vi "Block_No_Av.vi"(2 "Desired Averaging Time (mins)":dbl=5.0, 3 "Raw data file":path, 4 "Results file":path) -> ()   [LabVIEW 2022 SP3]
uses:
  Controls/Post_Process.ctl
  Controls/Setup.ctl
  Controls/Save_Data.ctl
  Globals/Meas_global.vi
  Block_Control_global.vi
  Globals/Dynamic_call_global.ph.vi
panel:
  out "Current Row Number":i32
  out "No of Rows":i32
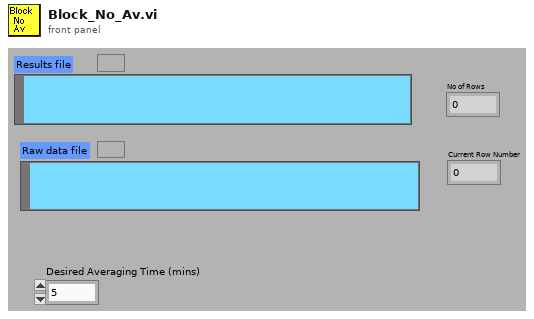
[diagram p1: front panel]
types:
  T1 = typedef "Save_Data.ctl" = enum16{"Save No Data", "Save Data"}
  T2 = typedef "Setup.ctl" = enum16{"Run Program", "Show Setup", "Save Current Setup", "Setup Front Panel"}
  T3 = typedef "Post_Process.ctl" = enum16{"Take New Data", "Post Process Raw Data File"}
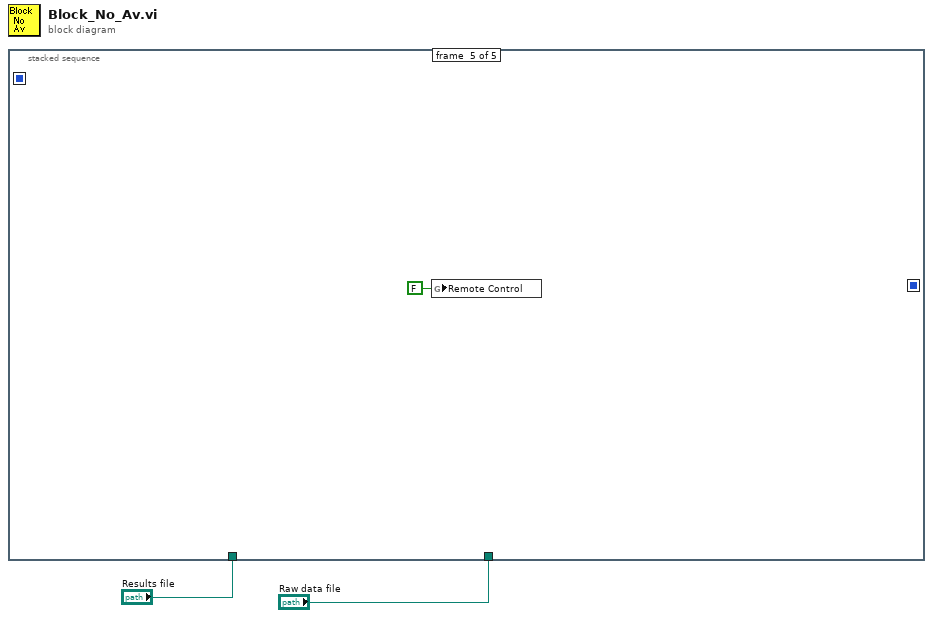
[diagram p0: block diagram]
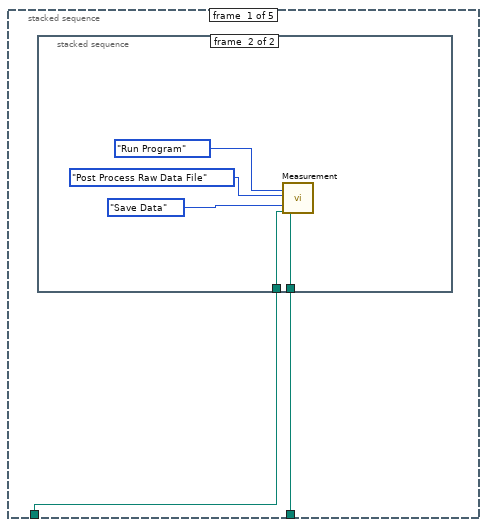
[diagram p2: hidden frame]
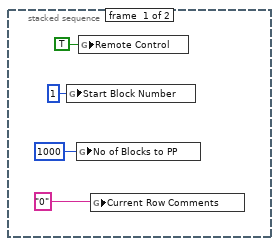
[diagram p3: hidden frame]
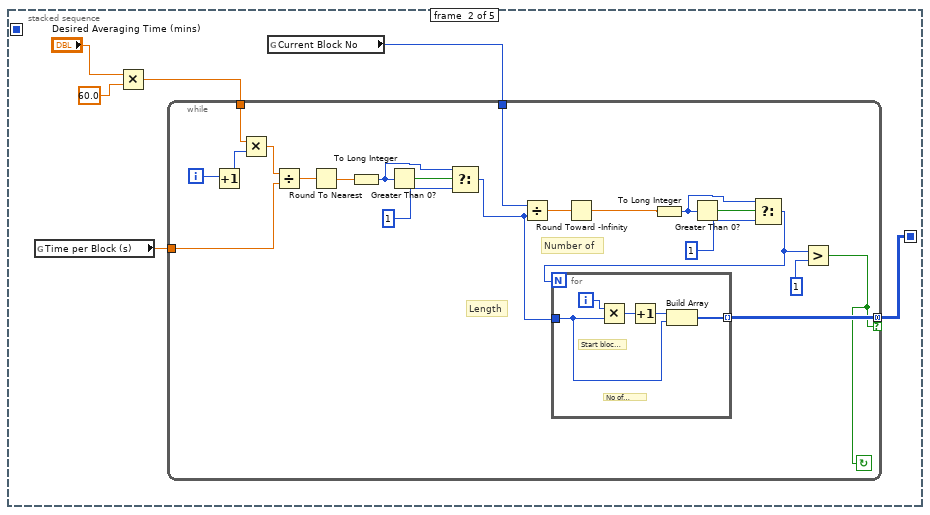
[diagram p4: hidden frame]
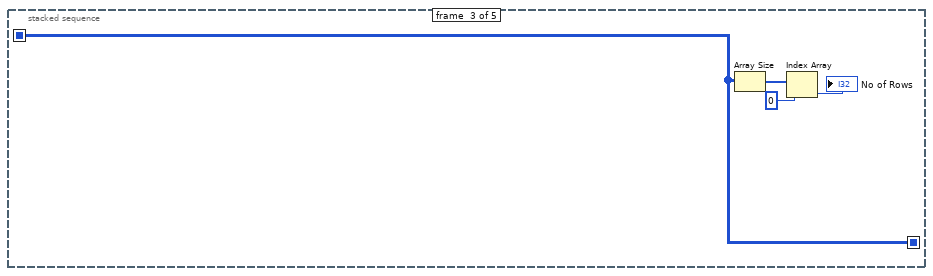
[diagram p5: hidden frame]
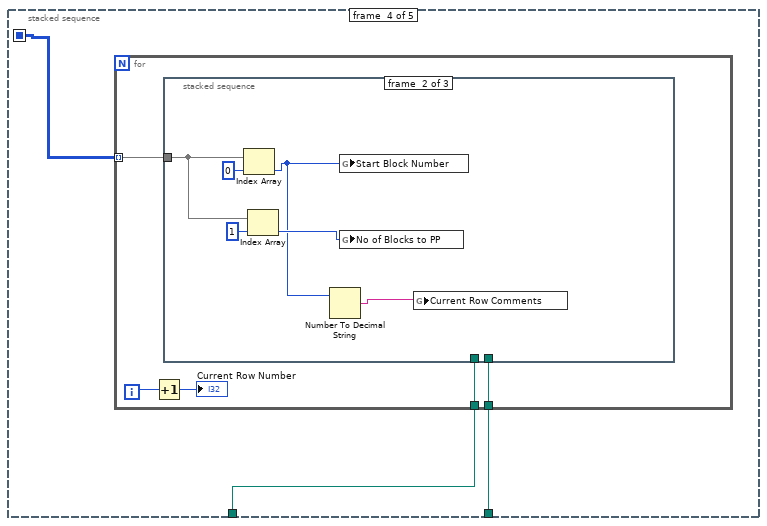
[diagram p6: hidden frame]
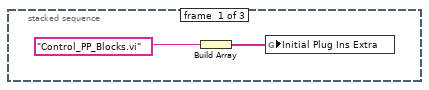
[diagram p7: hidden frame]
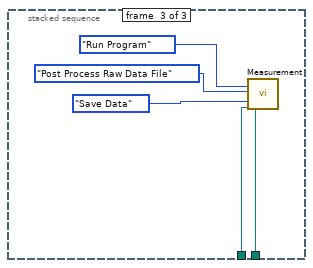
[diagram p8: hidden frame]
diagram:
  n1 = stacked-sequence {
    seq-local: [_ _ w46 _ _] -> [_ _ _ w50 _]
    seq-local: [_ w14 _ _ _] -> [_ _ w46 _ _]
    tunnel: "Raw data file" -> [w4 _ _ w52 _]
    tunnel: "Results file" -> [w3 _ _ w51 _]
    frame #0 {
      n2 = stacked-sequence {
        tunnel: w4 -> [_ w11]
        tunnel: w3 -> [_ w10]
        frame #0 {
          n3 = global write "Block_Control_global.vi" "Start Block Number"(1 ("Start Block Number")) -> ()
          n4 = global write "Block_Control_global.vi" "No of Blocks to PP"(1000 ("Start Block Number")) -> ()
          n5 = global write "Block_Control_global.vi" "Remote Control"(TRUE ("Remote Control")) -> ()
          n6 = global write "Meas_global.vi" "Current Row Comments"("0") -> ()
        }
        frame #1 {
          n7 = call "Measurement.vi"("setup"=Setup."Run Program", "Post Process"=Post_Process."Post Process Raw Data File", "File"=Save_Data."Save Data", "Results file"=w10, "Raw data file"=w11) -> ()  [unwired: 1 in, 14 out]
        }
      }
    }
    frame #1 {
      n8 = global read "Meas_global.vi" "Time per Block (s)"() -> (w18:dbl)
      n9 = Multiply(x="Desired Averaging Time (mins)", y=60.0) -> (x*y=w15:dbl)
      n10 = global read "Meas_global.vi" "Current Block No"() -> (w19:i32)
      n11 = while {
        tunnel: w19 -> [w40]
        tunnel: w18 -> [w26]
        tunnel: w15 -> [w25]
        tunnel: [w21] -> w14 mode=concatenating if=w20
        i -> [w28]
        stop <- w20 continue-if-true
        # "Length"
        # "Number of"
        n12 = Increment(x=w28) -> (x+1=w27:i32)
        n13 = Multiply(x=w25, y=w27) -> (x*y=w24:dbl)
        n14 = Divide(x=w24, y=w26) -> (x/y=w38:dbl)
        n15 = Round To Nearest(number=w38) -> (nearest integer value=w37:dbl)
        n16 = To Long Integer(number=w37) -> (32bit integer=w35:i32)
        n17 = Greater Than 0?(x=w35) -> (x > 0?=w36:bool)
        n18 = Select(t=w35, s=w36, f=1) -> (s? t:f=w29:i32)
        n19 = Divide(x=w40, y=w29) -> (x/y=w39:dbl)
        n20 = Round Toward -Infinity(1:w39) -> (0:w30:dbl)
        n21 = To Long Integer(number=w30) -> (32bit integer=w32:i32)
        n22 = Greater Than 0?(x=w32) -> (x > 0?=w31:bool)
        n23 = Select(t=w32, s=w31, f=1) -> (s? t:f=w23:i32)
        n24 = for {
          N: w23 -> [_]
          tunnel: [w45] -> w21 mode=indexing
          tunnel: w29 -> [w41]
          i -> [w43]
          # "Start block No"
          # "No of blocks"
          n25 = Multiply(x=w43, y=w41) -> (x*y=w44:i32)
          n26 = Increment(x=w44) -> (x+1=w42:i32)
          n27 = Build Array(w42, w41) -> (w45:i32[])
        }
        n28 = Greater?(x=w23, y=1) -> (0:w20:bool)
      }
    }
    frame #2 {
      n29 = Array Size(array=w46) -> (size(s)=w49:i32[])
      n30 = Index Array(array=w49, index=0) -> (element=→"No of Rows":i32)
    }
    frame #3 {
      n31 = for {
        tunnel: w52 -> [w57]
        tunnel: w51 -> [w56]
        tunnel: w50 -> [w55] mode=indexing
        i -> [w54]
        n32 = Increment(x=w54) -> (x+1=→"Current Row Number":i32)
        n33 = stacked-sequence {
          tunnel: w57 -> [_ _ w68]
          tunnel: w56 -> [_ _ w67]
          tunnel: w55 -> [_ w63 _]
          frame #0 {
            n34 = Build Array("Control_PP_Blocks.vi") -> (w58:string[])
            n35 = global write "Dynamic_call_global.ph.vi" "Initial Plug Ins Extra"(w58) -> ()
          }
          frame #1 {
            n36 = Index Array(array=w63, index=0) -> (element=w61:i32)
            n37 = Index Array(array=w63, index=1) -> (element=w62:i32)
            n38 = Number To Decimal String(number=w61) -> (decimal integer string=w60:string)  [unwired: 1 in]
            n39 = global write "Block_Control_global.vi" "Start Block Number"(w61) -> ()
            n40 = global write "Block_Control_global.vi" "No of Blocks to PP"(w62) -> ()
            n41 = global write "Meas_global.vi" "Current Row Comments"(w60) -> ()
          }
          frame #2 {
            n42 = call "Measurement.vi"("setup"=Setup."Run Program", "Post Process"=Post_Process."Post Process Raw Data File", "File"=Save_Data."Save Data", "Results file"=w67, "Raw data file"=w68) -> ()  [unwired: 1 in, 14 out]
          }
        }
      }
    }
    frame #4 {
      n43 = global write "Block_Control_global.vi" "Remote Control"(FALSE ("Remote Control")) -> ()
    }
  }
